vi "check_start_conditions.vi"(6 "stop at FIFO overflow?":bool, 7 "FIFO overflow?":bool, 8 "Bidirectional acquisition":bool, 9 "FPGA Scan Counters":T1={"Current part of waveform"=2, "Current waveform"=0} {"Current part of waveform" items=["Imaging", "Settling", "Resting"]}, 10 "wait for trigger?":bool, 11 "Scan":bool) -> (1 "Scanning?":bool, 2 "acquire?":bool)   [LabVIEW 2011]
uses:
  typedefs/scan_counters_cluster.ctl
  <vilib>/rvi/eio/common/nirviEmuTemplateMethod_errors.vi
  <vilib>/eio/EIONode/EIONode.xnode
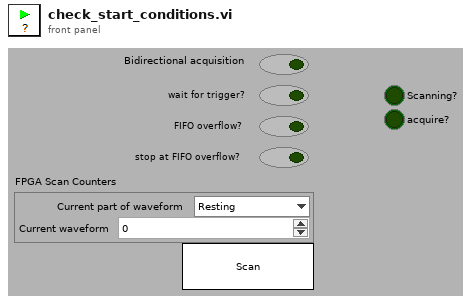
[diagram p1: front panel]
types:
  T1 = typedef "scan_counters_cluster.ctl" = cluster{"Current part of waveform":u8, "Current waveform":u16}
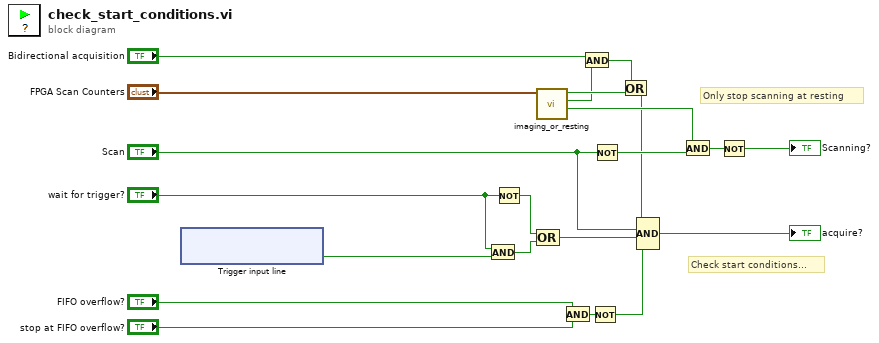
[diagram p0: block diagram]
diagram:
  # "Only stop scanning at resting"
  # "Check start conditions..."
  n1 = xnode "Trigger input line"() -> ("Connector0/DIO34"=w20:bool)  [unwired: 1 in, 1 out]
  n2 = And(x="wait for trigger?", y=w20) -> (x .and. y?=w18:bool)
  n3 = Not(x="wait for trigger?") -> (.not. x?=w21:bool)
  n4 = call "imaging_or_resting.vi"("Scan counters"="FPGA Scan Counters") -> ("Currently at resting part?"=w6:bool, "Currently at settling part?"=w2:bool, "Currently at imaging part?"=w4:bool)  [unwired: 8 in]
  n5 = Compound Arithmetic op=OR(w21, w18) -> (w14:bool)
  n6 = And(x="FIFO overflow?", y="stop at FIFO overflow?") -> (x .and. y?=w15:bool)
  n7 = And(x="Bidirectional acquisition", y=w2) -> (x .and. y?=w5:bool)
  n8 = Not(x=w15) -> (.not. x?=w13:bool)
  n9 = Not(x="Scan") -> (.not. x?=w10:bool)
  n10 = Or(x=w5, y=w4) -> (x .or. y?=w3:bool)
  n11 = Compound Arithmetic op=AND(w3, "Scan", w14, w13) -> (→"acquire?":bool)
  n12 = And(x=w6, y=w10) -> (x .and. y?=w9:bool)
  n13 = Not(x=w9) -> (.not. x?=→"Scanning?":bool)
